vi "AOTF laser control manual.vi"(6 "DAQ setup":enum16{"Test setup", "Microscope"}(ring), 11 "Laser Toggles":T1 {"Laser 642 nm power" min=0.0 max=5.0 scale=0.0..100.0; "Laser 595 nm power" min=0.0 max=5.0 scale=0.0..100.0; "Laser 560 nm power" min=0.0 max=5.0 scale=0.0..100.0; "Laser 488 nm power" min=0.0 max=5.0 scale=0.0..100.0}) -> ()   [LabVIEW 2020]
uses:
  typedefs/Laser_toggles__manual_typedef.ctl
  <vilib>/DAQmx/write.llb/DAQmx Write (Digital 1D Bool NChan 1Samp 1Line).vi
  <vilib>/DAQmx/create/channels.llb/DAQmx Create Channel (DO-Digital Output).vi
  <vilib>/DAQmx/miscellaneous.llb/DAQmx Fill In Error Info.vi
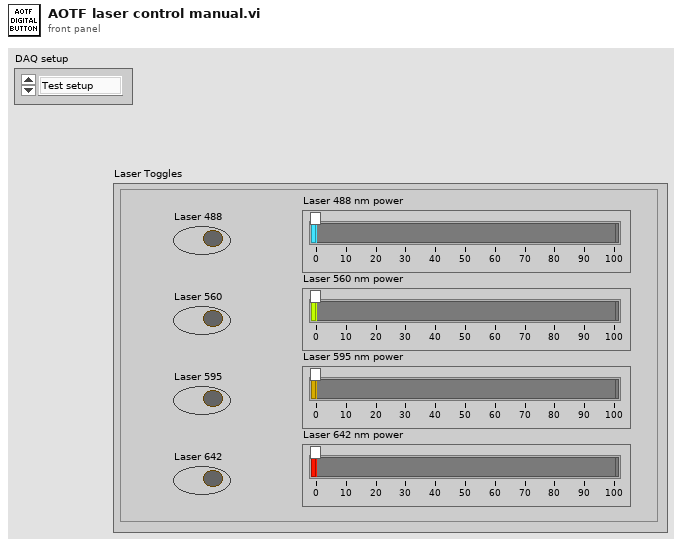
[diagram p1: front panel]
types:
  T1 = typedef "Laser_toggles__manual_typedef.ctl" = cluster{"Laser 488 nm power":dbl, "Laser 560 nm power":dbl, "Laser 595 nm power":dbl, "Laser 642 nm power":dbl, "Laser 560 ":bool, "Laser 595 ":bool, "Laser 642 ":bool, "Laser 488 ":bool}
  T2 = typedef "DAQ_channel_typedef.ctl" = cluster{"CO.Pulse.Term":tag, "Voice coil analog output":tag, "counter":tag, "CO.Pulse.Term 2":tag, "AOTF lines":tag, "counter 2":tag, "CO.Pulse.Term 3":tag, "counter 3":tag}
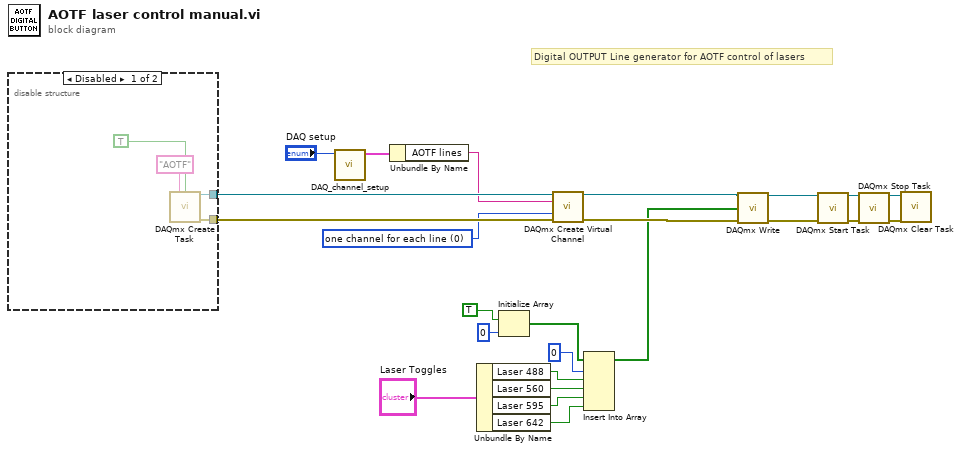
[diagram p0: block diagram]
diagram:
  w14 = 0 items=["one channel for each line", "one channel for all lines"] ("line grouping")
  # "Digital OUTPUT Line generator for AOTF control of lasers"
  n1 = disable-structure shown="Disabled" {
    disable-tunnel: [w27 _] -> w22
    disable-tunnel: [w26 _] -> w21
    frame Disabled {
      n2 = call <vilib>:"DAQmx Create Task.vi"("new task name"="AOTF", "auto cleanup"=TRUE) -> ("task out"=w27:refnum<k21>, "error out"=w26:errorcluster)  [unwired: 12 in]
    }
    frame Enabled {
    }
  }
  n3 = call "DAQ_channel_setup.vi"("Text Ring"="DAQ setup") -> ("DAQ channels OUT"=w2:T2)  [unwired: 10 in]
  n4 = Unbundle By Name(w2) -> ("AOTF lines"=w1:tag)
  n5 = Unbundle By Name("Laser Toggles") -> ("Laser 488"=w9:bool, "Laser 560"=w8:bool, "Laser 595"=w7:bool, "Laser 642"=w6:bool)
  n6 = Initialize Array(TRUE, 0 ("dimension size")) -> (w10:bool[])
  n7 = call-poly <vilib>:"DAQmx Create Virtual Channel.vi"("task in"=w22, "lines"=w1, "line grouping"=w14, "error in"=w21) -> ("task out"=w20:refnum<k21>, "error out"=w19:errorcluster)  [unwired: 10 in]
  n8 = Insert Into Array(array=w10, index=0, new element #1=w9, new element #2=w8, new element #3=w7, new element #4=w6) -> (w5:bool[])
  n9 = call-poly <vilib>:"DAQmx Write.vi"("task/channels in"=w20, "data"=w5, "error in"=w19) -> ("task out"=w24:refnum<k21>, "error out"=w23:errorcluster)  [unwired: 10 in, 1 out]
  n10 = call <vilib>:"DAQmx Start Task.vi"("task/channels in"=w24, "error in"=w23) -> ("task out"=w16:refnum<k21>, "error out"=w15:errorcluster)  [unwired: 12 in]
  n11 = call <vilib>:"DAQmx Stop Task.vi"("task/channels in"=w16, "error in"=w15) -> ("task out"=w18:refnum<k21>, "error out"=w17:errorcluster)  [unwired: 12 in]
  n12 = call <vilib>:"DAQmx Clear Task.vi"("task in"=w18, "error in"=w17) -> ()  [unwired: 13 in, 1 out]
